vi "read_list.vi"(8 "error in (no error)":errorcluster, 11 "StringList in":refnum<class "StringList.lvclass">) -> (0 "error out":errorcluster, 2 "List Items":string[](array[string]), 3 "StringList out":refnum<class "StringList.lvclass">)   [LabVIEW 2015, in "StringList.lvlib" / "StringList.lvclass"]
uses:
  StringList.lvclass
  StringList.lvclass/StringList.ctl
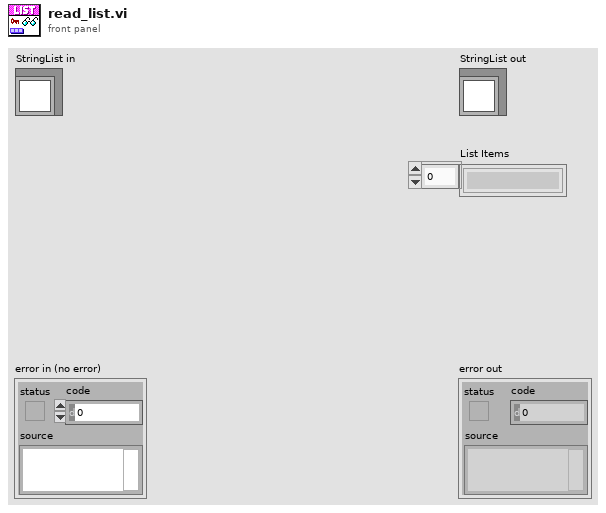
[diagram p1: front panel]
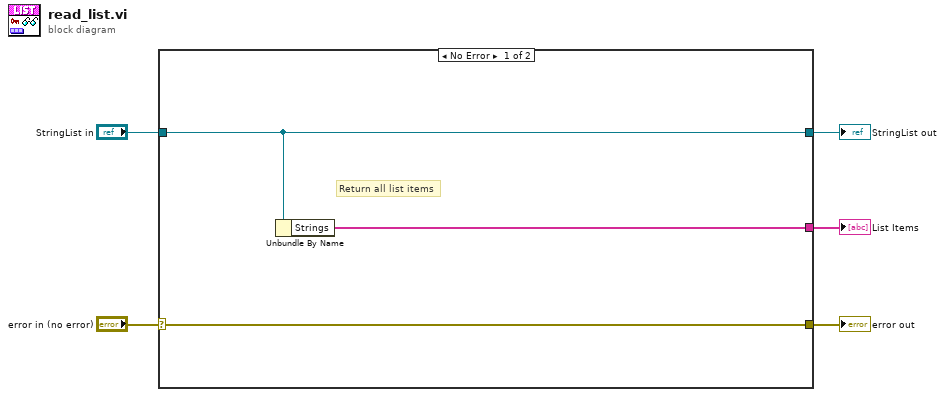
[diagram p0: block diagram]
diagram:
  n1 = case shown="No Error" "error in (no error)" {
    selector: "error in (no error)" -> [w8 w10]
    tunnel: [w8 w10] -> w4
    tunnel: [w7 w9] -> w2
    tunnel: "StringList in" -> [w7 w9]
    tunnel: [w6 _] -> w1
    frame No Error {
      # "Return all list items"
      n2 = Unbundle By Name(w7) -> ("Strings"=w6:string[])
    }
    frame Error {
    }
  }
  "error out" <- w4
  "StringList out" <- w2
  "List Items" <- w1
